vi "EEC EST 300 Editing Steps Within a File.vi"(7 "Internal scanner?":bool, 8 "error in (no error)":errorcluster, 10 "DCW Test Parameters (in)":T2={"Voltage (0~6.0 KV)"=1.0, "High Limit(0.0~7500 uA)"=0.0, "Low Limit(0~7500 uA)"=0.0, "Ramp Up Time (0.1~999.9 seconds)"=0.4, "Dwell Time (0, 0.4~999.9 seconds)"=1.0, "Ramp Down Time (0, 1.0~999.9 seconds)"=0.0, "Charge LO (0.0~350uA)"=0.0, "Arc Sense (1~9)"=5, "Arc Detect (F: Off)"=FALSE, "Auto Charge LO (F: Off)"=FALSE, "Ramp-Hi (0.0~7500 uA)"=0.0} {"Ramp-Hi (0.0~7500 uA)" format="%.2f"; "Ramp Down Time (0, 1.0~999.9 seconds)" format="%.1f"; "Charge LO (0.0~350uA)" format="%.2f"; "Dwell Time (0, 0.4~999.9 seconds)" format="%.1f"; "Ramp Up Time (0.1~999.9 seconds)" format="%.1f"; "Low Limit(0~7500 uA)" format="%.1f"; "High Limit(0.0~7500 uA)" format="%.1f"}, 11 "VISA resource name":refnum<visa-resource-name>) -> (0 "error out":errorcluster, 1 "error Occured?":bool, 2 "Number of Steps (0)":i32, 3 "Step Parameters":string)   [LabVIEW 2020]
doc: "This VI is an example of how to edit steps. This will take previously created file \"RandomT\" and edit the DCW parameters.\nNOTE: \"Creating and Saving a File\" is required to run before this VI."
uses:
  <instrlib>/eec EST 300/Public/Configure/Steps/Low Level/DCW Test Parameters.ctl
  <instrlib>/eec EST 300/Public/Configure/Steps/Low Level/Scanner Settings.ctl
  <instrlib>/eec EST 300/eec EST 300.lvlib
panel:
  in  "Scanner Settings":T1={"Scan1"=1, "Scan2"=1, "Scan3"=1, "Scan4"=1, "Scan5"=1, "Scan6"=1, "Scan7"=1, "Scan8"=1, "Scan9"=1, "Scan10"=1, "Scan11"=1, "Scan12"=1, "Scan13"=1, "Scan14"=1, "Scan15"=1, "Scan16"=1} {"Scan16" scale=0.0..2.0; "Scan15" scale=0.0..2.0; "Scan14" scale=0.0..2.0; "Scan13" scale=0.0..2.0; "Scan12" scale=0.0..2.0; "Scan11" scale=0.0..2.0; "Scan10" scale=0.0..2.0; "Scan9" scale=0.0..2.0; "Scan8" scale=0.0..2.0; "Scan7" scale=0.0..2.0; "Scan6" scale=0.0..2.0; "Scan5" scale=0.0..2.0; "Scan4" scale=0.0..2.0; "Scan3" min=0 max=2 scale=0.0..2.0; "Scan2" min=0 max=2 scale=0.0..2.0; "Scan1" min=0 max=2 scale=0.0..2.0}
  # "On\nOff"
  # "On\nOff"
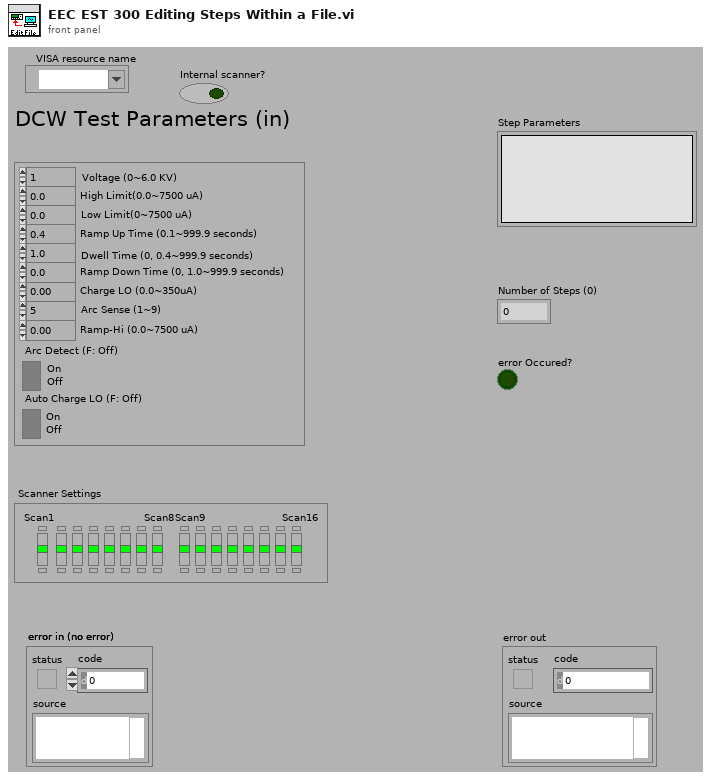
[diagram p1: front panel]
types:
  T1 = typedef "EEC EST 300.lvlib/Scanner Settings.ctl" = cluster{"Scan1":i32, "Scan2":i32, "Scan3":i32, "Scan4":i32, "Scan5":i32, "Scan6":i32, "Scan7":i32, "Scan8":i32, "Scan9":i32, "Scan10":i32, "Scan11":i32, "Scan12":i32, "Scan13":i32, "Scan14":i32, "Scan15":i32, "Scan16":i32}
  T2 = typedef "eec EST 300.lvlib/DCW Test Parameters.ctl" = cluster{"Voltage (0~6.0 KV)":dbl, "High Limit(0.0~7500 uA)":dbl, "Low Limit(0~7500 uA)":dbl, "Ramp Up Time (0.1~999.9 seconds)":dbl, "Dwell Time (0, 0.4~999.9 seconds)":dbl, "Ramp Down Time (0, 1.0~999.9 seconds)":dbl, "Charge LO (0.0~350uA)":dbl, "Arc Sense (1~9)":i32, "Arc Detect (F: Off)":bool, "Auto Charge LO (F: Off)":bool, "Ramp-Hi (0.0~7500 uA)":dbl}
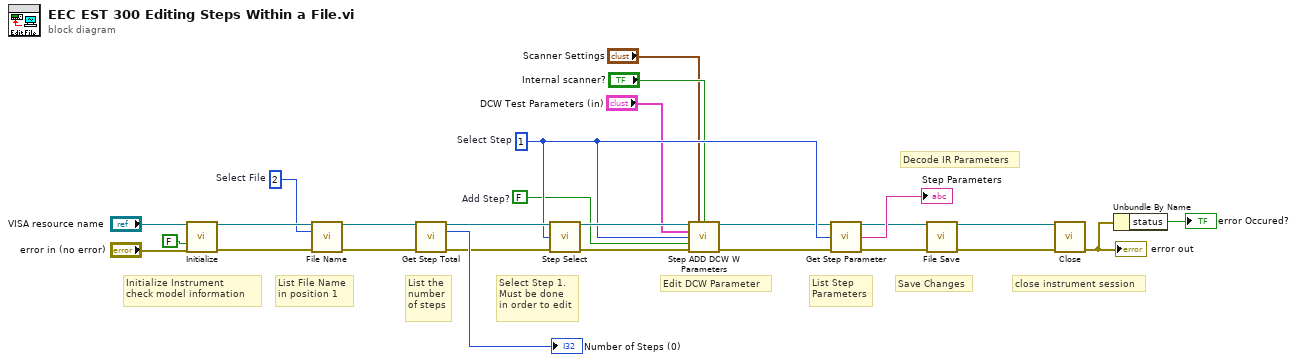
[diagram p0: block diagram]
diagram:
  w8 = 1  # Select Step
  w7 = FALSE  # Add Step?
  w20 = 2  # Select File
  # "Save Changes"
  # "List Step\nParameters"
  # "Edit DCW Parameter"
  # "Select Step 1.\nMust be done\nin order to edit"
  # "List the\nnumber\nof steps"
  # "close instrument session"
  # "Decode IR Parameters"
  # "List File Name\nin position 1"
  # "Initialize Instrument \ncheck model information"
  n1 = call <instrlib>:"Initialize.vi"("VISA resource name"="VISA resource name", "Reset (True)"=FALSE, "error in (no error)"="error in (no error)") -> ("VISA resource name out"=w22:refnum<visa-resource-name>, "error out"=w21:errorcluster)  [unwired: 10 in, 1 out]
  n2 = call <instrlib>:"File Name.vi"("VISA resource name"=w22, "File Number"=w20, "error in (no error)"=w21) -> ("VISA resource name out"=w19:refnum<visa-resource-name>, "error out"=w18:errorcluster)  [unwired: 10 in, 1 out]
  n3 = call <instrlib>:"Get Step Total.vi"("VISA resource name"=w19, "error in (no error)"=w18) -> ("VISA resource name out"=w13:refnum<visa-resource-name>, "# of Steps"=→"Number of Steps (0)":i32, "error out"=w12:errorcluster)  [unwired: 11 in]
  n4 = call <instrlib>:"Step Select.vi"("VISA resource name"=w13, "Step Number (1)"=w8, "error in (no error)"=w12) -> ("VISA resource name out"=w9:refnum<visa-resource-name>, "error out"=w6:errorcluster)  [unwired: 11 in]
  n5 = call <instrlib>:"Step ADD DCW W Parameters.vi"("VISA resource name"=w9, "Scanner Settings"="Scanner Settings", "Internal scanner?"="Internal scanner?", "DCW Test Parameters (in)"="DCW Test Parameters (in)", "Step Selection (1-200)"=w8, "Add Step"=w7, "error in (no error)"=w6) -> ("VISA resource name out"=w4:refnum<visa-resource-name>, "error out"=w3:errorcluster)  [unwired: 7 in]
  n6 = call <instrlib>:"Get Step Parameter.vi"("VISA resource name"=w4, "Step Number (0 = Active Step)"=w8, "error in (no error)"=w3) -> ("VISA resource name out"=w11:refnum<visa-resource-name>, "Step Parameter"=→"Step Parameters":string, "error out"=w10:errorcluster)  [unwired: 10 in]
  n7 = call <instrlib>:"File Save.vi"("VISA resource name"=w11, "error in (no error)"=w10) -> ("VISA resource name out"=w16:refnum<visa-resource-name>, "error out"=w17:errorcluster)  [unwired: 12 in]
  n8 = call <instrlib>:"Close.vi"("VISA resource name"=w16, "error in (no error)"=w17) -> ("error out"=w23:errorcluster)  [unwired: 13 in]
  "error out" <- w23
  n9 = Unbundle By Name(w23) -> ("status"=→"error Occured?":bool)
